vi "BlockDiagramPath.vi"(0 "GObj Refnum":refnum<vi>, 11 "error in (no error)":errorcluster) -> (4 "UID[]":string[](array[string]), 6 "ClassName[]":string[](array[string]), 8 "Reference[]":refnum<vi>[](array[refnum]), 15 "error out":errorcluster)   [LabVIEW 2016, in "LabVIEWCodeCoverage.lvlib"]
uses:
  LabVIEWCodeCoverage.lvlib
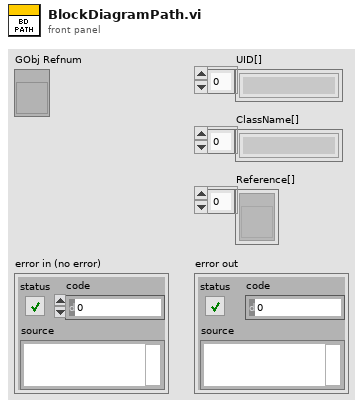
[diagram p1: front panel]
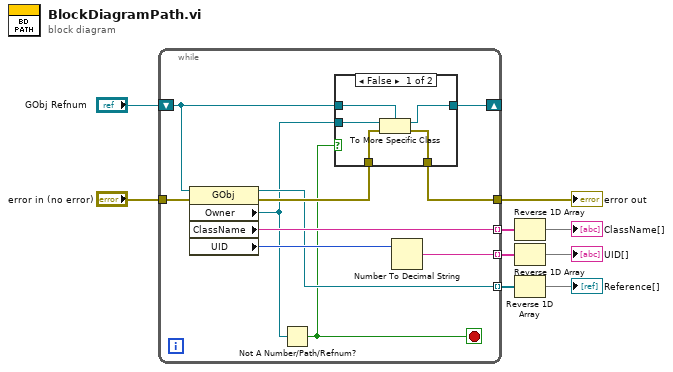
[diagram p0: block diagram]
diagram:
  n1 = while {
    tunnel: "error in (no error)" -> [w20]
    tunnel: [w18] -> w5 mode=indexing
    tunnel: [w17] -> w6 mode=indexing
    tunnel: [w16] -> w7
    shift-right: [w13] -> _
    shift-left: "GObj Refnum" -> [w14]
    tunnel: [w12] -> w2 mode=indexing
    stop <- w10 stop-if-true
    n2 = property class="GObj"(reference=w14, error in=w20) -> (reference out=w12:refnum<vi>, error out=w15:errorcluster, "Owner"=w11:refnum<vi>, "ClassName"=w17:string, "UID"=w19:i32)
    n3 = Not A Number/Path/Refnum?(number/path/refnum=w11) -> (NaN/Path/Refnum?=w10:bool)
    n4 = case shown="False" w10 {
      tunnel: [w25 w27] -> w16
      tunnel: w15 -> [w24 w27]
      tunnel: w14 -> [w23 w26]
      tunnel: [w22 w26] -> w13
      tunnel: w11 -> [w21 _]
      frame False {
        n5 = To More Specific Class(target class=w23, reference=w21, error in=w24) -> (specific class reference=w22:refnum<vi>, error out=w25:errorcluster)
      }
      frame True {
      }
    }
    n6 = Number To Decimal String(number=w19) -> (decimal integer string=w18:string)  [unwired: 1 in]
  }
  "error out" <- w7
  n7 = Reverse 1D Array(array=w6) -> (reversed array=→"ClassName[]":string[])
  n8 = Reverse 1D Array(array=w5) -> (reversed array=→"UID[]":string[])
  n9 = Reverse 1D Array(array=w2) -> (reversed array=→"Reference[]":refnum<vi>[])
